vi "CMD_POTLINE.vi"(6 "Gantry in":refnum<class "Gantry Class.lvclass">, 8 "error in (no error)":errorcluster, 10 "Arguments":string[](array[string]), 11 "gScript Interpreter in":refnum<class "gScript Interpreter.lvclass">) -> (0 "error out":errorcluster, 3 "gScript Interpreter out":refnum<class "gScript Interpreter.lvclass">, 4 "Gantry out":refnum<class "Gantry Class.lvclass">)   [LabVIEW 2017, in "gScript Interpreter.lvclass"]
uses:
  gScript Interpreter.lvclass
  Shared Components/Gantry Class/Gantry Class.lvclass
  Shared Components/SyringeTool Class/SyringeTool Class.lvclass
  C:/Users/cfang/Desktop/pixel-gantry-control/Gantry/Shared Components/Gantry Class/Gantry Class.lvclass
  <vilib>/Utility/error.llb/Error Cluster From Error Code.vi
  <vilib>/ErrorRing/Error Ring.xnode
  Shared Components/FlexWorktable/FlexWorktable.lvclass
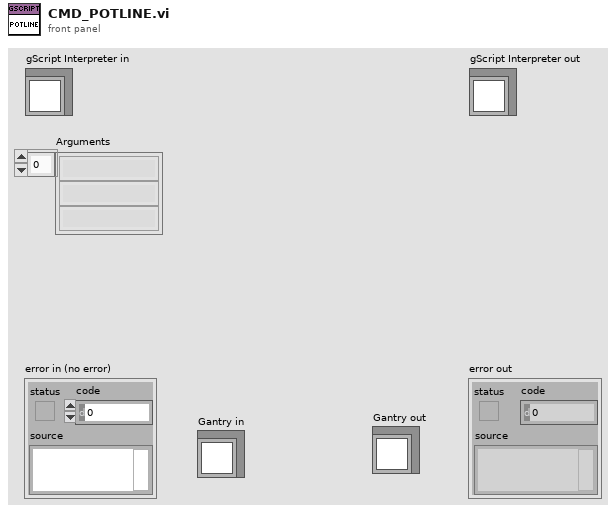
[diagram p1: front panel]
types:
  T1 = typedef "Memory Cell.ctl" = cluster{"type":T2, "x":dbl, "y":dbl, "z":dbl, "w":dbl}
  T2 = typedef "Memory Cell Type Enum.ctl" = enum16{"integer", "float", "vector", "rotation"}
  T3 = cluster{"Syringe Holder":string, "Mixing Time":timestamp, "Tip Offset":refnum<class "Vec3d Class.lvclass">}
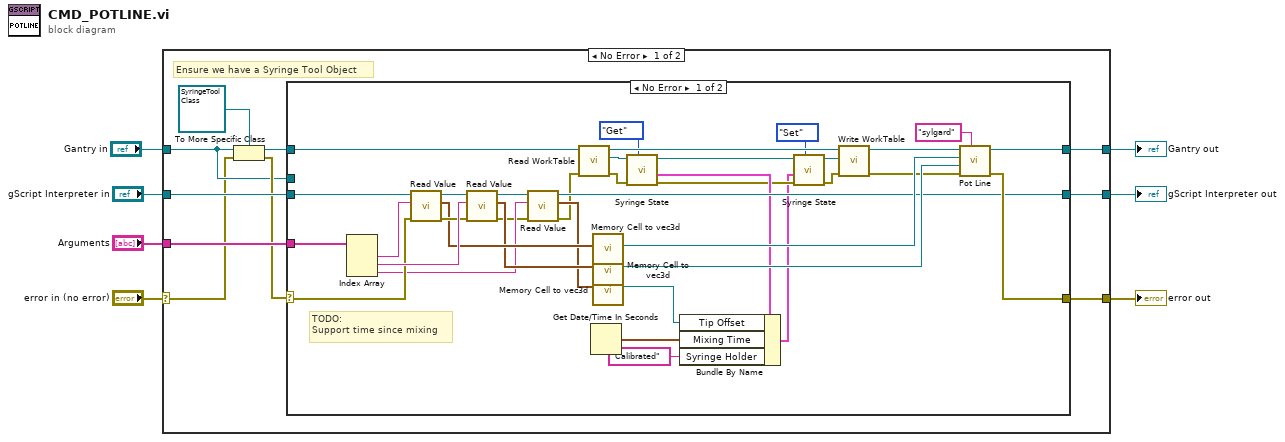
[diagram p0: block diagram]
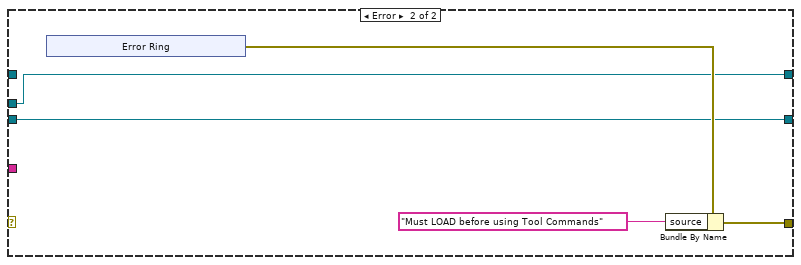
[diagram p2: hidden frame]
diagram:
  n1 = case shown="No Error" "error in (no error)" {
    selector: "error in (no error)" -> [w8 w66]
    tunnel: [w13 w66] -> w6
    tunnel: [w15 w65] -> w4
    tunnel: "gScript Interpreter in" -> [w16 w65]
    tunnel: "Arguments" -> [w17 _]
    tunnel: "Gantry in" -> [w9 w64]
    tunnel: [w14 w64] -> w1
    frame No Error {
      # "Ensure we have a Syringe Tool Object"
      n2 = To More Specific Class(target class=refnum<class "SyringeTool Class.lvclass"> refnum ("SyringeTool out"), reference=w9, error in=w8) -> (specific class reference=w10:refnum<class "SyringeTool Class.lvclass">, error out=w11:errorcluster)
      n3 = case shown="No Error" w11 {
        selector: w11 -> [w42 _]
        tunnel: w17 -> [w54 _]
        tunnel: w16 -> [w53 w56]
        tunnel: [w32 w56] -> w15
        tunnel: [w44 w55] -> w14
        tunnel: [w43 w57] -> w13
        tunnel: w10 -> [w41 _]
        tunnel: w9 -> [_ w55]
        frame No Error {
          # "TODO:\nSupport time since mixing"
          n4 = Index Array(array=w54) -> (element #1=w52:string, element #2=w50:string, element #3=w37:string)  [unwired: 3 in]
          n5 = call-dynamic "Read Value.vi"("error in (no error)"=w42, "String in"=w52, "gScript Interpreter in"=w53) -> ("error out"=w49:errorcluster, "Memory Cell"=w48:T1, "gScript Interpreter out"=w51:refnum<class "gScript Interpreter.lvclass">)  [unwired: 6 in]
          n6 = call-dynamic "Read Value.vi"("error in (no error)"=w49, "String in"=w50, "gScript Interpreter in"=w51) -> ("error out"=w33:errorcluster, "Memory Cell"=w47:T1, "gScript Interpreter out"=w38:refnum<class "gScript Interpreter.lvclass">)  [unwired: 6 in]
          n7 = call-dynamic "Read Value.vi"("error in (no error)"=w33, "String in"=w37, "gScript Interpreter in"=w38) -> ("error out"=w21:errorcluster, "Memory Cell"=w36:T1, "gScript Interpreter out"=w32:refnum<class "gScript Interpreter.lvclass">)  [unwired: 6 in]
          n8 = call-dynamic "Read WorkTable.vi"("error in"=w21, "Gantry Class in"=w41) -> ("error out"=w20:errorcluster, "Worktable"=w30:refnum<class "FlexWorktable.lvclass">, "Gantry Class out"=w40:refnum<class "SyringeTool Class.lvclass">)  [unwired: 7 in]
          n9 = Get Date/Time In Seconds() -> (seconds since 1Jan1904=w34:timestamp)
          n10 = call "Memory Cell to vec3d.vi"("Memory Cell"=w48) -> ("Vec3d out"=w46:refnum<class "Vec3d Class.lvclass">)  [unwired: 10 in]
          n11 = call "Memory Cell to vec3d.vi"("Memory Cell"=w47) -> ("Vec3d out"=w45:refnum<class "Vec3d Class.lvclass">)  [unwired: 10 in]
          n12 = call "Memory Cell to vec3d.vi"("Memory Cell"=w36) -> ("Vec3d out"=w35:refnum<class "Vec3d Class.lvclass">)  [unwired: 10 in]
          n13 = call-dynamic "Syringe State.vi"("Get/Set"=enum16{"Get", "Set"}."Get", "error in (no error)"=w20, "FlexWorktable in"=w30) -> ("error out"=w24:errorcluster, "Syringe out"=w28:T3, "FlexWorktable out"=w27:refnum<class "FlexWorktable.lvclass">)  [unwired: 6 in]
          n14 = Bundle By Name(cluster=w28, "Tip Offset"=w35, "Mixing Time"=w34, "Syringe Holder"="Calibrated") -> (w19:T3)
          n15 = call-dynamic "Syringe State.vi"("Get/Set"=enum16{"Get", "Set"}."Set", "error in (no error)"=w24, "Syringe in"=w19, "FlexWorktable in"=w27) -> ("error out"=w23:errorcluster, "FlexWorktable out"=w26:refnum<class "FlexWorktable.lvclass">)  [unwired: 5 in, 1 out]
          n16 = call-dynamic "Write WorkTable.vi"("error in (no error)"=w23, "FlexWorktable"=w26, "Gantry Class in"=w40) -> ("error out"=w22:errorcluster, "Gantry Class out"=w39:refnum<class "SyringeTool Class.lvclass">)  [unwired: 7 in]
          n17 = call-dynamic "Pot Line.vi"("Encapsulant"="sylgard", "error in"=w22, "End Position"=w45, "Start Position"=w46, "SyringeTool in"=w39) -> ("error out"=w43:errorcluster, "SyringeTool out"=w44:refnum<class "SyringeTool Class.lvclass">)  [unwired: 5 in]
        }
        frame Error {
          n18 = xnode "Error Ring"() -> ("error out"=w59:errorcluster)
          n19 = Bundle By Name(cluster=w59, "source"="Must LOAD before using Tool Commands") -> (w57:errorcluster)
        }
      }
    }
    frame Error {
    }
  }
  "error out" <- w6
  "gScript Interpreter out" <- w4
  "Gantry out" <- w1
